vi "TEMPConfigure Dialog.vi"(8 "error in (no error)":errorcluster, 11 "Message in":refnum<class "Message.lvclass">) -> (0 "error out":errorcluster, 2 "Ok?":bool, 3 "Message out":refnum<class "Message.lvclass">)   [LabVIEW 2015, in "Dialog Template.lvclass"]
uses:
  Dialog Template.lvclass
  <vilib>/ActorFramework/Message/Message.lvclass
panel:
  in  "Cancel Button":bool
  in  "OK Button":bool
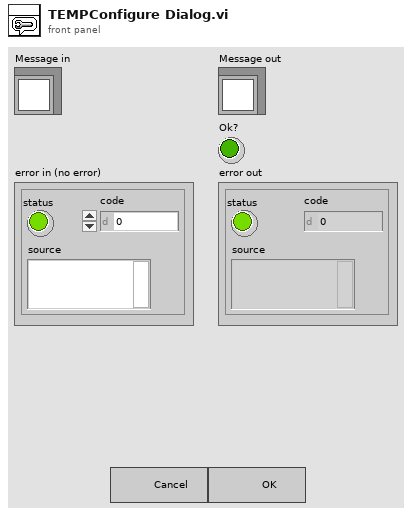
[diagram p1: front panel]
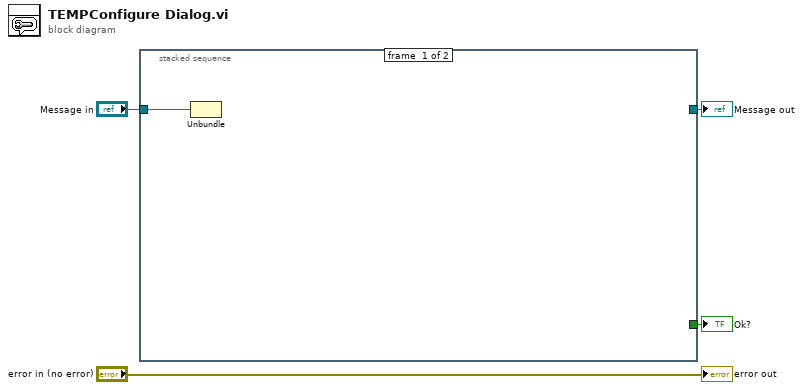
[diagram p0: block diagram]
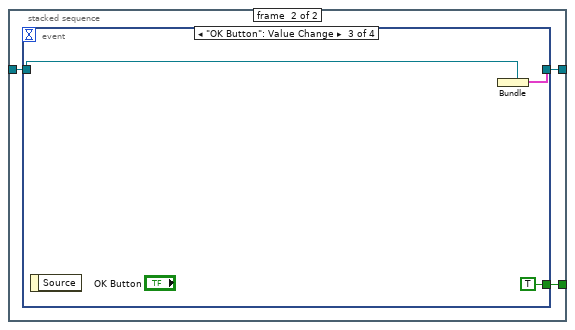
[diagram p2: hidden frame]
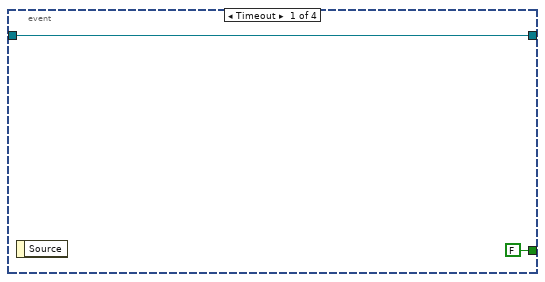
[diagram p3: hidden frame]
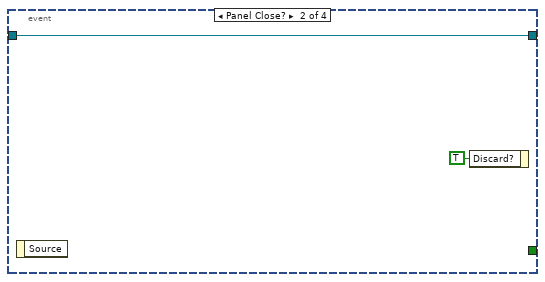
[diagram p4: hidden frame]
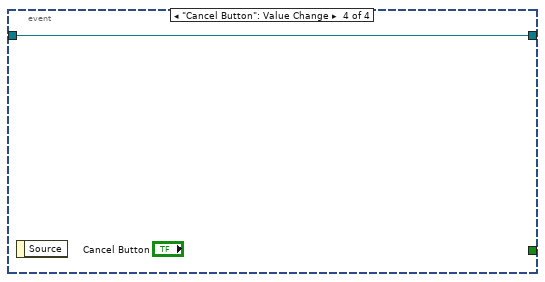
[diagram p5: hidden frame]
diagram:
  n1 = stacked-sequence {
    tunnel: [_ w8] -> w3
    tunnel: [_ w7] -> w2
    tunnel: "Message in" -> [w5 w6]
    frame #0 {
      n2 = Unbundle ("Seq0Unbundler")(w5) -> ()  [unwired: 2 out]
    }
    frame #1 {
      n3 = event shown="[2] \"OK Button\": Value Change" {
        selector: _ -> [_ _ _ _]
        dyn-events: _ -> [_ _ _ _]
        timeout: _ -> [_ _ _ _]
        tunnel: [w9 w11 w13 w16] -> w7
        tunnel: w6 -> [w9 w11 w15 w16]
        tunnel: [FALSE _ TRUE _] -> w8
        event Timeout {
          n4 = event-data() -> ()  [unwired: 1 in, 1 out]
        }
        event Panel Close? {
          n5 = event-data() -> ()  [unwired: 1 in, 1 out]
          n6 = event-data("Discard?"=TRUE) -> ()  [unwired: 1 in, 1 out]
        }
        event "OK Button": Value Change {
          n7 = event-data() -> ()  [unwired: 1 in, 1 out]
          n8 = Bundle ("Main-Bundler")(cluster=w15) -> (w13:cluster{void})  [unwired: 1 in]
        }
        event "Cancel Button": Value Change {
          n9 = event-data() -> ()  [unwired: 1 in, 1 out]
        }
      }
    }
  }
  "Ok?" <- w3
  "Message out" <- w2
  "error out" <- "error in (no error)"
